vi "_034.vi"() -> ()   [LabVIEW 2024]
panel:
  out "Array":dbl[](array[numeric])
  out "s? t:f":string
  in  "Numeric":dbl
  out "sorted array":dbl[](array[numeric])
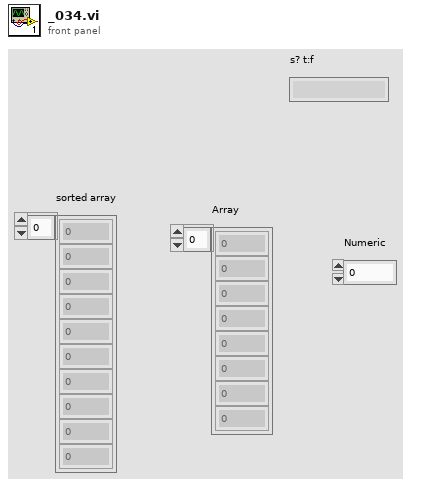
[diagram p1: front panel]
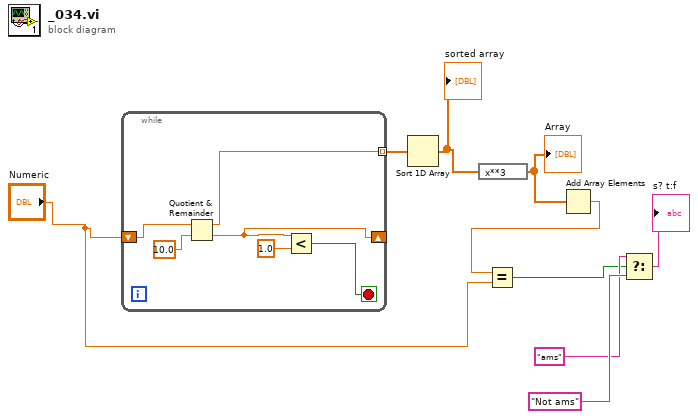
[diagram p0: block diagram]
diagram:
  n1 = while {
    shift-right: [w10] -> _
    shift-left: "Numeric" -> [w11]
    tunnel: [w12] -> w8 mode=indexing
    stop <- w13 stop-if-true
    n2 = Quotient & Remainder(x=w11, y=10.0) -> (x-y*floor(x/y)=w12:dbl, floor(x/y)=w10:dbl)
    n3 = Less?(x=w10, y=1.0) -> (x < y?=w13:bool)
  }
  n4 = Sort 1D Array(array=w8) -> (sorted array=w9:dbl[])
  "sorted array" <- w9
  n5 = expression code="x**3"(w9) -> (w2:dbl[])
  "Array" <- w2
  n6 = Add Array Elements(numeric array=w2) -> (sum=w4:dbl)
  n7 = Equal?(x=w4, y="Numeric") -> (x = y?=w1:bool)
  n8 = Select(t="ams", s=w1, f="Not ams") -> (s? t:f=→"s? t:f":string)
